vi "Fetch Multi-Point [MP].vi"(8 "error in (no error)":errorcluster, 9 "array size":i32, 10 "maximum time (5s)":dbl[unit]=5000.0, 11 "CS++DMM in":refnum<class "CS++DMM.lvclass">) -> (0 "error out":errorcluster, 1 "actual number of points":i32, 2 "reading array":dbl[](array[numeric]) format="%^.2e", 3 "CS++DMM out":refnum<class "CS++DMM.lvclass">)   [LabVIEW 2016, in "CS++DMM.lvlib" / "CS++DMM.lvclass"]
doc: "This VI returns an array of values from a previously initiated multi-point measurement. The number of measurements the DMM takes is determined by the values you specify for the Trigger Count and Sample Count parameters of the IviDmm Configure Multi-Point [MP] VI.\n\nYou must first call the IviDmm Initiate VI to initiate a measurement before calling this VI.\n\nNotes:\n\n(1) This VI is part of the IviDmmMultiPoint [MP] extension group.\n\n(2) After this VI executes, each element in the Reading Array parameter is an actual reading or a value indicating that an over-range condition occurred.\n\n(3) If an over-range condition occurs, the corresponding Reading Array element contains an IEEE defined NaN (Not a Number) value and the VI returns IVIDMM_WARN_OVER_RANGE (0x3FFA2001). \n\n(4) You can test each element in the Reading Array parameter for over-range with the IviDmm Is Over-Range VI.\n\n(5) The class driver returns a simulated measurement when this VI is called and the IviDmm>>Inherent IVI Settings>>User Options>>Simulate property is set to TRUE and the IviDmm>>Inherent IVI Settings>>User Options>>Use Specific Simulation property is set to FALSE. For information on how to configure a simulated measurement, refer to the online help manual.\n\n(6) This VI does not check the instrument status. Typically, you call this VI only in a sequence of calls to other low-level driver VIs. The sequence performs one operation. You use the low-level VIs to optimize one or more aspects of interaction with the instrument. If you want to check the instrument status, call the IviDmm Error-Query VI at the conclusion of the sequence."
uses:
  CS++DMM.lvclass
  CS++DMM.lvclass/CS++DMM.ctl
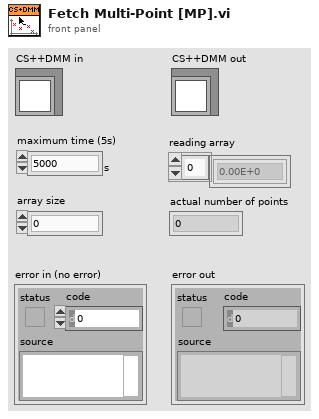
[diagram p1: front panel]
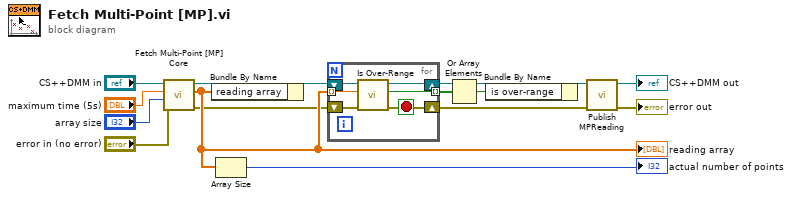
[diagram p0: block diagram]
diagram:
  n1 = call-dynamic "Fetch Multi-Point [MP] Core.vi"("error in (no error)"="error in (no error)", "array size"="array size", "maximum time (5s)"="maximum time (5s)", "CS++DMM in"="CS++DMM in") -> ("error out"=w3:errorcluster, "reading array"=w4:dbl[], "CS++DMM out"=w9:refnum<class "CS++DMM.lvclass">)  [unwired: 4 in, 1 out]
  "reading array" <- w4
  n2 = Bundle By Name(cluster=w9, "reading array"=w4) -> (w5:refnum<class "CS++DMM.lvclass">)
  n3 = Array Size(array=w4) -> (size(s)=→"actual number of points":i32)
  n4 = for {
    tunnel: [w22] -> w6 mode=indexing
    tunnel: w4 -> [w18] mode=indexing
    shift-right: [w19] -> w7
    shift-left: w5 -> [w20]
    shift-right: [w17] -> w2
    shift-left: w3 -> [w21]
    stop <- w17 stop-if-true
    n5 = call "Is Over-Range.vi"("error in (no error)"=w21, "measurement value"=w18, "CS++DMM in"=w20) -> ("error out"=w17:errorcluster, "is over-range"=w22:bool, "CS++DMM out"=w19:refnum<class "CS++DMM.lvclass">)  [unwired: 6 in]
  }
  n6 = Or Array Elements(Boolean array=w6) -> (logical OR=w8:bool)
  n7 = Bundle By Name(cluster=w7, "is over-range"=w8) -> (w1:refnum<class "CS++DMM.lvclass">)
  n8 = call "Publish MPReading.vi"("error in (no error)"=w2, "CS++DMM in"=w1) -> ("error out"=→"error out":errorcluster, "CS++DMM out"=→"CS++DMM out":refnum<class "CS++DMM.lvclass">)  [unwired: 8 in]
